vi "Destruct.vi"(8 "Error in (no error)":errorcluster, 11 "LogWriterDb in":refnum<class "LogWriterDb.lvclass">) -> (0 "Error out":errorcluster, 2 "Array log out":T1[](array[typedef]) {"Priority" items=["EMERGENCY", "ALERT", "CRITICAL", "ERROR", "WARNING", "NOTICE", "INFO", "DEBUG"]})   [LabVIEW 2011, in "LogWriterDb.lvclass"]
uses:
  LogWriterDb.lvclass
  Log/LogCluster.ctl
  Log/PrioritiesRing.ctl
  <vilib>/addons/database/Connection.llb/Conn ObjectReference.ctl
  <vilib>/addons/database/NI_Database_API.lvlib
  Log/Log.lvclass
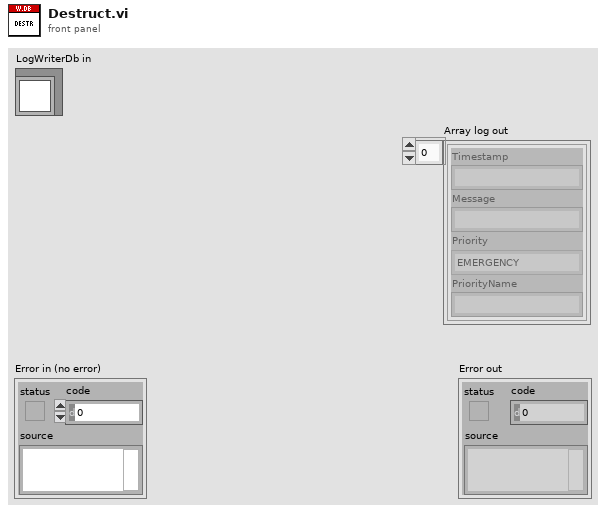
[diagram p1: front panel]
types:
  T1 = typedef "Log.lvclass/LogCluster.ctl" = cluster{"Timestamp":string, "Message":string, "Priority":T2, "PriorityName":string}
  T2 = typedef "Log.lvclass/PrioritiesRing.ctl" = u32
  T3 = typedef "NI_Database_API.lvlib/Conn ObjectReference.ctl" = refnum<k1>
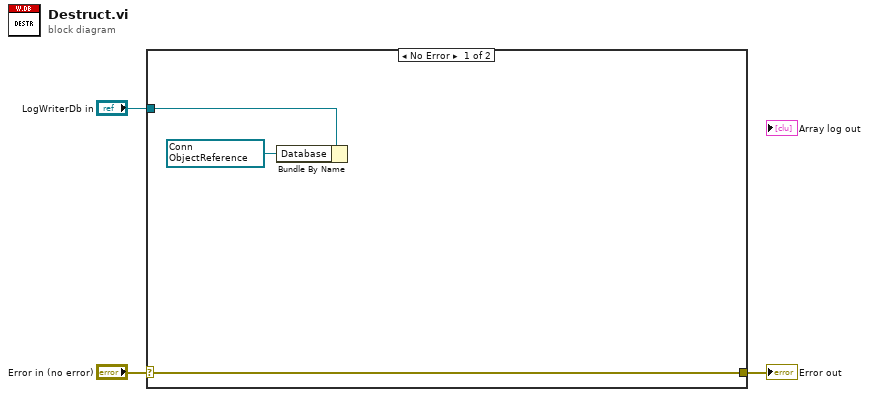
[diagram p0: block diagram]
diagram:
  n1 = case shown="No Error" "Error in (no error)" {
    selector: "Error in (no error)" -> [w6 w7]
    tunnel: [w6 w7] -> w2
    tunnel: "LogWriterDb in" -> [w5 _]
    frame No Error {
      w4 = T3 refnum items=["Connection"] ("Database")
      n2 = Bundle By Name(cluster=w5, "Database"=w4) -> ()  [unwired: 1 out]
    }
    frame Error {
    }
  }
  "Error out" <- w2
